vi "Frame.vi"(8 "error in (no error)":errorcluster, 11 "Node Ptr":T2 format="%.0x") -> (0 "error out":errorcluster)   [LabVIEW 2019, in "Diagnostics Addon System Explorer.lvlib"]
uses:
  Diagnostics Addon System Explorer.lvlib
  <vilib>/NI VeriStand/Custom Device API/Custom Device Item Ref.ctl
  Addon Shared/Types/Type.ctl
  Types/FG.Action.ctl
  SubVIs/Signal.FG.vi
  SubVIs/Frame.GetSignalRefs.vi
  Addon Shared/SubVIs/Constants.vi
  <vilib>/NI/NI VeriStand Advanced SysDef API/SysDef API/SysDef.Property.Set.vi
  <vilib>/NI/NI VeriStand Advanced SysDef API/_SubVIs/SysDef.Property.Set.U32.vi
  <vilib>/NI VeriStand/Custom Device API/NI VeriStand - Get Item Property.vi
  <vilib>/NI VeriStand/Custom Device API/Get Item Property (U32).vi
  <vilib>/NI VeriStand/Custom Device Tools/Custom Device Utility Library/NI VeriStand - Search for Item.vi
  <vilib>/NI VeriStand/Custom Device Tools/Custom Device Utility Library/NI VeriStand - Search for Item by GUID.vi
  <vilib>/NI VeriStand/Custom Device API/NI VeriStand - Get Item Children.vi
  <vilib>/NI/NI VeriStand Advanced SysDef API/_SubVIs/SysDef.Property.Set.DBL.vi
  <vilib>/NI/NI VeriStand Advanced SysDef API/_SubVIs/SysDef.Property.Set.String.vi
  <vilib>/NI VeriStand/Custom Device API/Get Item Property (Double).vi
  <vilib>/NI VeriStand/Custom Device API/Get Item Property (String).vi
  <vilib>/NI VeriStand/Custom Device API/NI VeriStand - Get Custom Device Channel Data.vi
  <vilib>/NI VeriStand/Custom Device API/Custom Device API.lvlib
  Addon Shared/Diagnostics Addon Shared.lvlib
panel:
  out "Type":T1
  out "Length":u32 caption="Length (bytes)"
  in  "ID":u16 format="%.0x"
  out "Signals":i32(listbox)
  in  "Description":string
  in  "Name":string
  in  "SHDocVw.IWebBrowser":refnum<k7>(container)
  in  "Header":cluster{"Section Name":string}={"Section Name"="Custom Device Item Settings"}
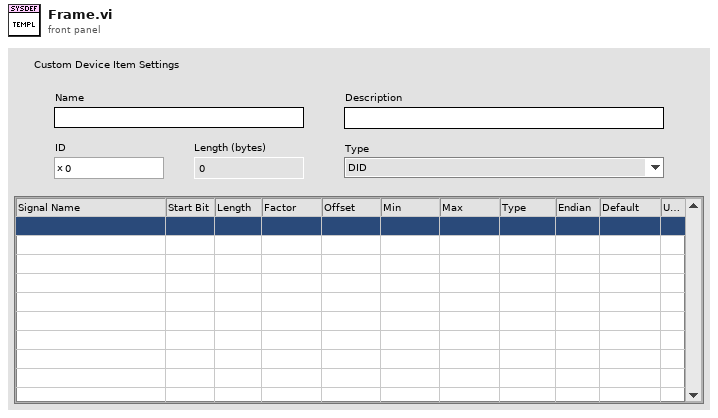
[diagram p1: front panel]
types:
  T1 = typedef "Diagnostics Addon Shared.lvlib/Type.ctl" = enum16{"DID", "CDID", "PID", "CPID", "Read Memory", "Write Memory", "IO Control", "Routine Start", "Routine Request", "Routine Stop", "User Defined", "DTC Control", "Clear DTCs", "Read DTCs", "Start DTCs", "DTC Change Count", "Tester Present", "Unlock ECU", "Reset ECU", "Diag Session Control", "Communication Control", "DPID Control", "Poll Control", "Diag CAN Control"}
  T2 = typedef "Custom Device API.lvlib/Custom Device Item Ref.ctl" = u64
  T3 = typedef "Diagnostics Addon System Explorer.lvlib/FG.Action.ctl" = enum16{"Get", "Set"}
  T4 = typedef "Custom Device API.lvlib/Custom Device Item Info.ctl" = cluster{"Name":string, "Is Channel":bool, "GUID":string, "Is Waveform":bool}
  T5 = typedef "Diagnostics Addon Shared.lvlib/Signal.ctl" = cluster{"Start Bit":u32, "Length":u32, "Scaling Factor":dbl, "Scaling Offset":dbl, "Minimum":dbl, "Maximum":dbl, "Data Type":u32, "Byte Order":u32, "Default Value":dbl, "Name":string, "Units":string}
  T6 = typedef "Custom Device API.lvlib/Custom Device Commands.ctl" = enum16{"Default", "Item renamed", "Shutdown", "Dynamic button pressed"}
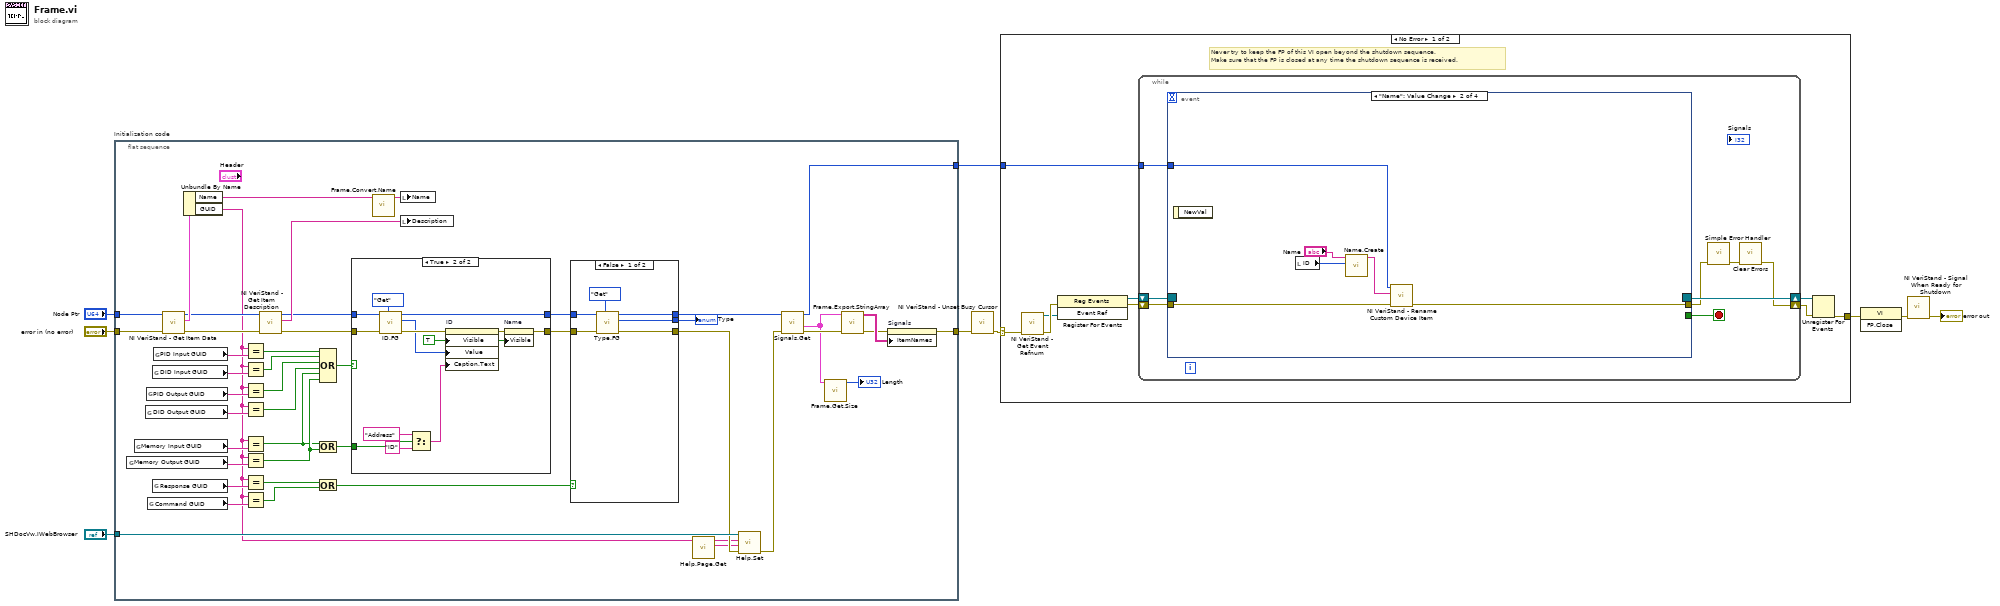
[diagram p0: block diagram]
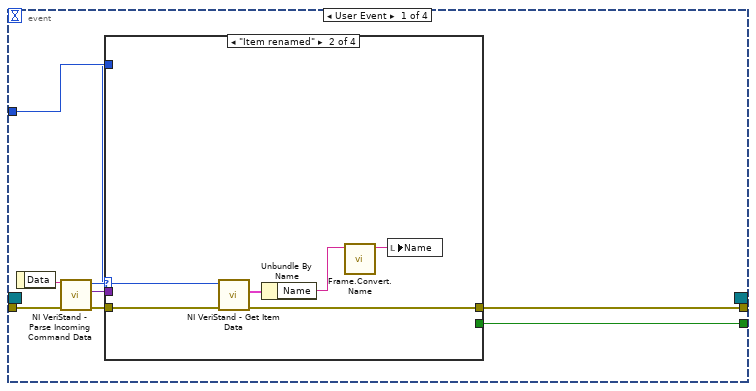
[diagram p2: hidden frame]
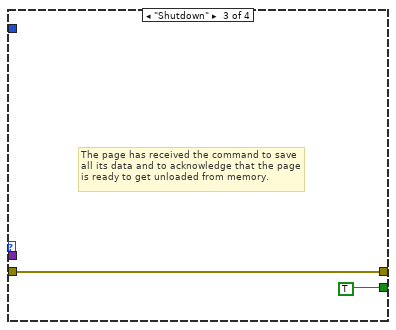
[diagram p4: hidden frame]
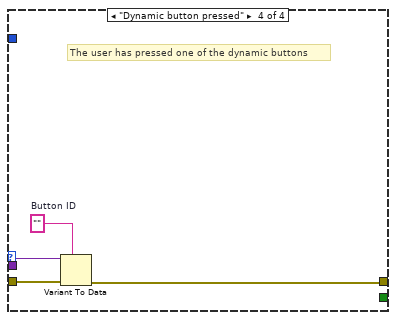
[diagram p5: hidden frame]
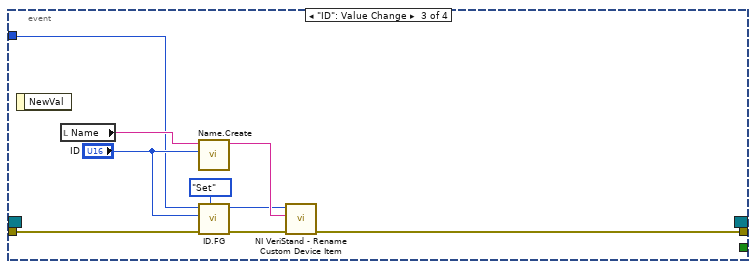
[diagram p6: hidden frame]
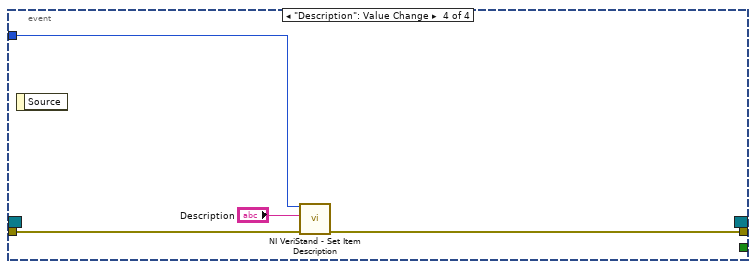
[diagram p7: hidden frame]
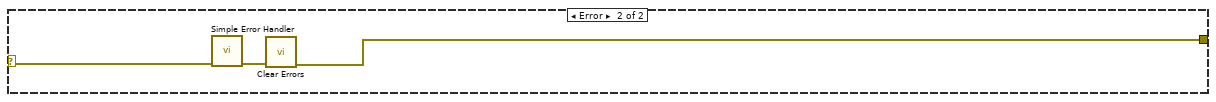
[diagram p8: hidden frame]
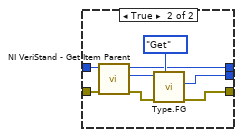
[diagram p9: hidden frame]
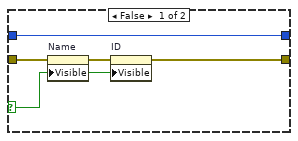
[diagram p10: hidden frame]
diagram:
  n1 = flat-sequence "Initialization code" {
    tunnel: "error in (no error)" -> [w43]
    tunnel: "Node Ptr" -> [w42]
    tunnel: [w53] -> w5
    tunnel: [w28] -> w2
    tunnel: "SHDocVw.IWebBrowser" -> [w41]
    frame #0 {
      n2 = global read "Constants.vi" "Memory Output GUID"() -> (w35:string)
      n3 = global read "Constants.vi" "Memory Input GUID"() -> (w34:string)
      n4 = global read "Constants.vi" "DID Output GUID"() -> (w33:string)
      n5 = global read "Constants.vi" "PID Output GUID"() -> (w32:string)
      n6 = global read "Constants.vi" "Command GUID"() -> (w24:string)
      n7 = global read "Constants.vi" "DID Input GUID"() -> (w39:string)
      n8 = global read "Constants.vi" "Response GUID"() -> (w13:string)
      n9 = global read "Constants.vi" "PID Input GUID"() -> (w47:string)
      n10 = call <vilib>:"NI VeriStand - Get Item Data.vi"("error in (no error)"=w43, "Item Ref in"=w42) -> ("error out"=w44:errorcluster, "Item Info"=w54:T4, "Item Ref out"=w45:T2)  [unwired: 7 out]
      n11 = Unbundle By Name(w54) -> ("Name"=w49:string, "GUID"=w10:string)
      n12 = Equal?(x=w10, y=w47) -> (x = y?=w46:bool)
      n13 = Equal?(x=w10, y=w39) -> (x = y?=w38:bool)
      n14 = Equal?(x=w10, y=w32) -> (x = y?=w29:bool)
      n15 = Equal?(x=w10, y=w33) -> (x = y?=w25:bool)
      n16 = Equal?(x=w10, y=w34) -> (x = y?=w30:bool)
      n17 = Equal?(x=w10, y=w35) -> (x = y?=w31:bool)
      n18 = Equal?(x=w10, y=w13) -> (x = y?=w14:bool)
      n19 = Equal?(x=w10, y=w24) -> (x = y?=w15:bool)
      n20 = call <vilib>:"NI VeriStand - Get Item Description.vi"("error in (no error)"=w44, "Item Ref in"=w45) -> ("error out"=w27:errorcluster, "Description"=w55:string, "Item Ref out"=w26:T2)  [unwired: 7 out]
      n21 = Compound Arithmetic op=OR(w46, w38, w29, w25, w30, w31) -> (w22:bool)
      n22 = Compound Arithmetic op=OR(w30, w31) -> (w23:bool)
      n23 = Compound Arithmetic op=OR(w14, w15) -> (w17:bool)
      n24 = case shown="True" w22 {
        selector: w22 -> [w72 _]
        tunnel: [w71 w76] -> w20
        tunnel: [w70 w75] -> w21
        tunnel: w27 -> [w73 w86]
        tunnel: w26 -> [w70 w85]
        tunnel: w23 -> [_ w80]
        frame False {
          n25 = property on="Name" class="Str"(error in=w73, "Visible"=w72) -> (error out=w74:errorcluster)  [unwired: 1 in, 1 out]
          n26 = property on="ID" class="DigNum (strict)"(error in=w74, "Visible"=w72) -> (error out=w71:errorcluster)  [unwired: 1 in, 1 out]
        }
        frame True {
          w81 = TRUE ("Visible")
          n27 = call "ID.FG.vi"("Action"=FG.Action."Get", "error in (no error)"=w86, "Device Item Ref in"=w85) -> ("error out"=w84:errorcluster, "ID"=w83:u32, "Device Item Ref out"=w75:T2)  [unwired: 6 in]
          n28 = Select(t="Address", s=w80, f="ID") -> (s? t:f=w77:string)
          n29 = property on="ID" class="DigNum (strict)"(error in=w84, "Visible"=w81, "Value"=w83, "Caption.Text"=w77) -> (error out=w82:errorcluster)  [unwired: 1 in, 1 out]
          n30 = property on="Name" class="Str"(error in=w82, "Visible"=w81) -> (error out=w76:errorcluster)  [unwired: 1 in, 1 out]
        }
      }
      n31 = call "Frame.Convert.Name.vi"("VS Frame Name"=w49) -> ("Frame Name"=w48:string)  [unwired: 9 in, 1 out]
      n32 = local write "Name"(w48) -> ()
      n33 = local write "Description"(w55) -> ()
      n34 = case shown="False" w17 {
        tunnel: w21 -> [w59 w66]
        tunnel: w20 -> [w60 w65]
        tunnel: [w58 w64] -> w19
        tunnel: [w57 w63] -> w18
        tunnel: [w56 w62] -> w16
        frame False {
          n35 = call "Type.FG.vi"("Action"=FG.Action."Get", "error in (no error)"=w60, "Device Item Ref in"=w59) -> ("error out"=w58:errorcluster, "Type"=w56:T1, "Device Item Ref out"=w57:T2)  [unwired: 6 in]
        }
        frame True {
          n36 = call <vilib>:"NI VeriStand - Get Item Parent.vi"("error in (no error)"=w65, "Item Ref in"=w66) -> ("error out"=w68:errorcluster, "Parent Ref"=w67:T2, "Item Ref out"=w63:T2)  [unwired: 6 in, 1 out]
          n37 = call "Type.FG.vi"("Action"=FG.Action."Get", "error in (no error)"=w68, "Device Item Ref in"=w67) -> ("error out"=w64:errorcluster, "Type"=w62:T1)  [unwired: 6 in, 1 out]
        }
      }
      "Type" <- w16
      n38 = call "Help.Page.Get.vi"("GUID"=w10) -> ("HTML File"=w11:string, "Main CHM File"=w12:string)  [unwired: 9 in]
      n39 = call "Help.Set.vi"("error in (no error)"=w19, "HTML File"=w11, "Main CHM File"=w12, "SHDocVw.IWebBrowser2"=w41) -> ("error out"=w40:errorcluster)  [unwired: 7 in]
      n40 = call "Signals.Get.vi"("error in (no error)"=w40, "Device Item Ref out"=w18) -> ("error out"=w51:errorcluster, "Parameters"=w37:T5[], "Item Ref out"=w28:T2)  [unwired: 6 in, 1 out]
      n41 = call "Frame.Get.Size.vi"("Parameters"=w37) -> ("Bytes"=→"Length":u32)  [unwired: 10 in]
      n42 = call "Frame.Export.StringArray.vi"("error in (no error)"=w51, "Frame Parameters"=w37) -> ("error out"=w50:errorcluster, "Frame Parameters"=w52:string[][])  [unwired: 8 in]
      n43 = property on="Signals" class="MCListbox (strict)"(error in=w50, "ItemNames"=w52) -> (error out=w53:errorcluster)  [unwired: 1 in, 1 out]
    }
  }
  n44 = call <vilib>:"NI VeriStand - Unset Busy Cursor.vi"("error in (no error)"=w5) -> ("error out"=w4:errorcluster)  [unwired: 10 out]
  n45 = case shown="No Error" w4 {
    selector: w4 -> [w88 w147]
    tunnel: [w93 w145] -> w9
    tunnel: w2 -> [w89 _]
    frame No Error {
      # "Never try to keep the FP of this VI open beyond the shutdown sequence.\nMake sure that the FP is closed at any time the shutdown sequence is received."
      n46 = call <vilib>:"NI VeriStand - Get Event Refnum.vi"("error in (no error)"=w88) -> ("error out"=w96:errorcluster, "Event Ref"=w92:refnum<user-event>)  [unwired: 9 out]
      n47 = register-events(error in=w96, w92) -> (reference out=w90:refnum<event-registration>, error out=w91:errorcluster)  [unwired: 1 in]
      n48 = while {
        tunnel: w89 -> [w100]
        shift-right: [w97] -> w94
        shift-left: w91 -> [w103]
        shift-right: [w104] -> w95
        shift-left: w90 -> [w102]
        stop <- w101 stop-if-true
        n49 = event shown="[1] \"Name\": Value Change" {
          selector: w102 -> [_ _ _ _]
          dyn-events: [_ _ _ _] -> w104
          timeout: _ -> [_ _ _ _]
          tunnel: w103 -> [w112 w131 w137 w143]
          tunnel: [w108 _ _ _] -> w101
          tunnel: [w107 w130 w139 w142] -> w99
          tunnel: w100 -> [w106 w129 w134 w144]
          event User Event {
            n50 = event-data() -> ("Data"=w111:string)  [unwired: 1 out]
            n51 = call <vilib>:"NI VeriStand - Parse Incoming Command Data.vi"("error in (no error)"=w112, "Incoming data"=w111) -> ("error out"=w110:errorcluster, "Outgoing data"=w105:variant, "Action"=w109:T6)  [unwired: 7 out]
            n52 = case shown="\"Item renamed\"" w109 {
              tunnel: w110 -> [w113 w119 w120 w125]
              tunnel: [_ _ TRUE _] -> w108
              tunnel: [w113 w116 w120 w122] -> w107
              tunnel: w106 -> [_ w118 _ _]
              tunnel: w105 -> [_ _ _ w124]
              frame "Default", Default {
              }
              frame "Item renamed" {
                n53 = call <vilib>:"NI VeriStand - Get Item Data.vi"("error in (no error)"=w119, "Item Ref in"=w118) -> ("error out"=w116:errorcluster, "Item Info"=w117:T4)  [unwired: 8 out]
                n54 = Unbundle By Name(w117) -> ("Name"=w115:string)
                n55 = call "Frame.Convert.Name.vi"("VS Frame Name"=w115) -> ("Frame Name"=w114:string)  [unwired: 9 in, 1 out]
                n56 = local write "Name"(w114) -> ()
              }
              frame "Shutdown" {
                # "The page has received the command to save all its data and to acknowledge that the page is ready to get unloaded from memory."
              }
              frame "Dynamic button pressed" {
                w123 = ""  # Button ID
                # "The user has pressed one of the dynamic buttons"
                n57 = Variant To Data(error in=w125, type=w123, Variant=w124) -> (error out=w122:errorcluster)  [unwired: 1 out]
              }
            }
          }
          event "Name": Value Change {
            n58 = event-data() -> ()  [unwired: 2 out]
            n59 = local read "ID"() -> (w128:u16)
            n60 = call "Name.Create.vi"("PID Number"=w128, "PID Name"="Name") -> ("VS Name"=w126:string)  [unwired: 9 in]
            n61 = call <vilib>:"NI VeriStand - Rename Custom Device Item.vi"("error in (no error)"=w131, "New Name"=w126, "Item Ref in"=w129) -> ("error out"=w130:errorcluster)  [unwired: 1 in, 7 out]
          }
          event "ID": Value Change {
            n62 = event-data() -> ()  [unwired: 2 out]
            n63 = local read "Name"() -> (w138:string)
            n64 = call "Name.Create.vi"("PID Number"="ID", "PID Name"=w138) -> ("VS Name"=w140:string)  [unwired: 9 in]
            n65 = call "ID.FG.vi"("Action"=FG.Action."Set", "error in (no error)"=w137, "ID"="ID", "Device Item Ref in"=w134) -> ("error out"=w136:errorcluster, "Device Item Ref out"=w133:T2)  [unwired: 5 in, 1 out]
            n66 = call <vilib>:"NI VeriStand - Rename Custom Device Item.vi"("error in (no error)"=w136, "New Name"=w140, "Item Ref in"=w133) -> ("error out"=w139:errorcluster)  [unwired: 1 in, 7 out]
          }
          event "Description": Value Change {
            n67 = event-data() -> ()  [unwired: 2 out]
            n68 = call <vilib>:"NI VeriStand - Set Item Description.vi"("error in (no error)"=w143, "Description"="Description", "Item Ref in"=w144) -> ("error out"=w142:errorcluster)  [unwired: 8 out]
          }
        }
        n69 = call <vilib>:"Simple Error Handler.vi"("error in (no error)"=w99) -> ("error out"=w98:errorcluster)  [unwired: 1 in, 7 out]
        n70 = call <vilib>:"Clear Errors.vi"("error in (no error)"=w98) -> ("error out"=w97:errorcluster)  [unwired: 1 in, 5 out]
      }
      n71 = Unregister For Events(event registration refnum=w95, error in=w94) -> (error out=w93:errorcluster)
    }
    frame Error {
      n72 = call <vilib>:"Simple Error Handler.vi"("error in (no error)"=w147) -> ("error out"=w146:errorcluster)  [unwired: 1 in, 7 out]
      n73 = call <vilib>:"Clear Errors.vi"("error in (no error)"=w146) -> ("error out"=w145:errorcluster)  [unwired: 1 in, 5 out]
    }
  }
  n74 = invoke class="VI" method="FP.Close"(error in=w9) -> (error out=w8:errorcluster)  [unwired: 2 in, 2 out]
  n75 = call <vilib>:"NI VeriStand - Signal When Ready for Shutdown.vi"("error in (no error)"=w8) -> ("error out"=→"error out":errorcluster)  [unwired: 10 out]
